vi "Modbus Master Example.vi"() -> ()   [LabVIEW 2016]
doc: "An example of the modbus master functionality."
uses:
  <vilib>/NI/Modbus Library/API/Master/Modbus Master.lvclass
  <vilib>/NI/Modbus Library/API/Wrapper/Create TCP Master.vi
  <vilib>/NI/Modbus Library/API/Wrapper/API Main.lvlib
panel:
  in  "Stop Button":bool
  in  "Port":u16=502
  in  "Set Holding Registers":bool
  in  "Fetch Input Registers":bool
  out "Status":string
  in  "Disconnect":bool
  in  "Connect":bool
  in  "Holding Registers":u16[](array[numeric])=[0, 0, 0, 0, 0, 0, 0, 0]
  out "Input Registers":u16[](array[numeric])
  in  "Slave Address":string="localhost"
  # "Input Registers are the integer inputs of a modbus device. This example allows you to read the first 8 inputs."
  # "Holding Registers are the integer outputs of a modbus device. This example allows you to set the first 8 outputs."
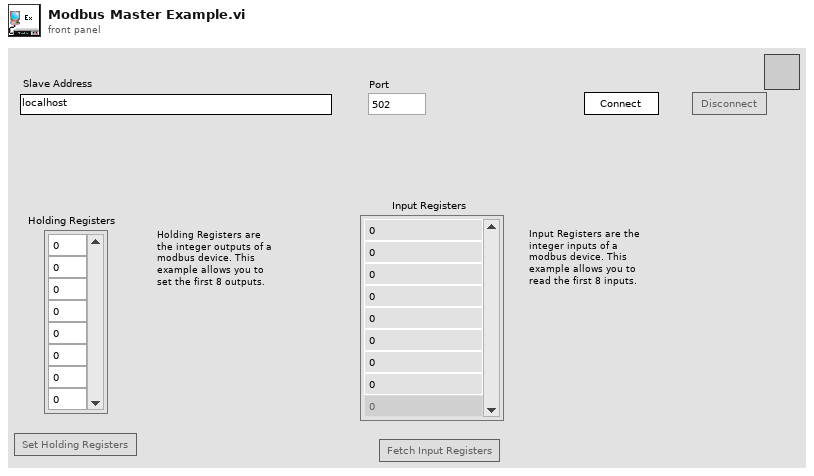
[diagram p1: front panel]
types:
  T1 = enum8{"Enabled", "Disabled", "Disabled and Grayed Out"}
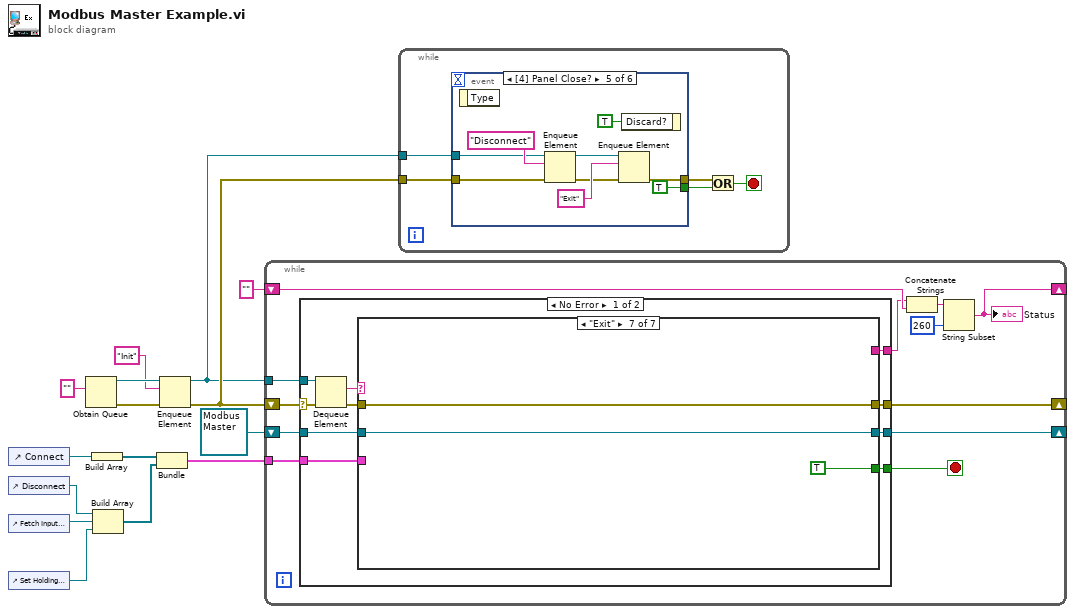
[diagram p0: block diagram]
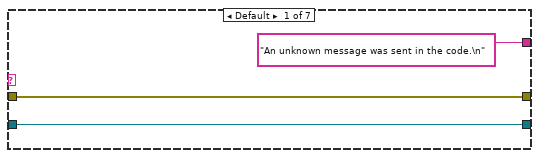
[diagram p2: hidden frame]
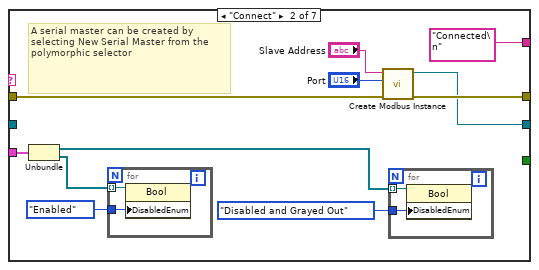
[diagram p3: hidden frame]
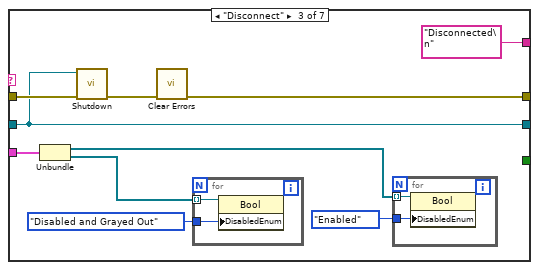
[diagram p4: hidden frame]
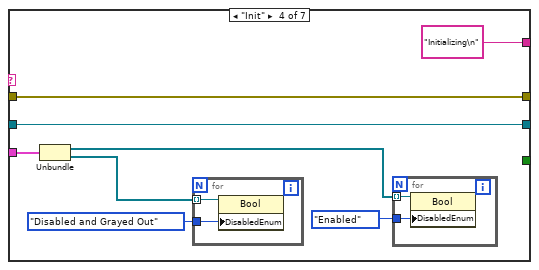
[diagram p5: hidden frame]
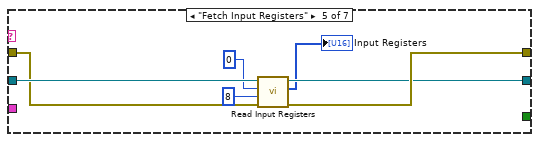
[diagram p6: hidden frame]
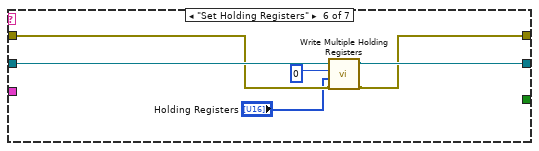
[diagram p7: hidden frame]
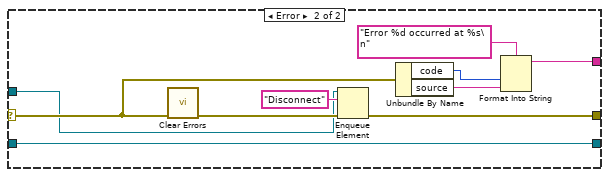
[diagram p8: hidden frame]
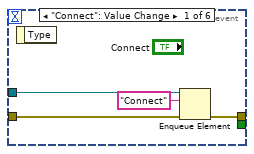
[diagram p9: hidden frame]
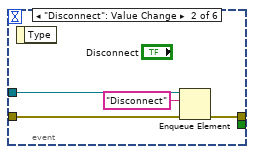
[diagram p10: hidden frame]
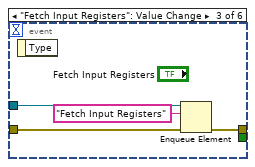
[diagram p11: hidden frame]
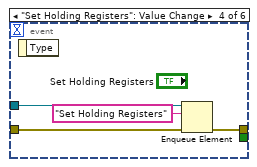
[diagram p12: hidden frame]
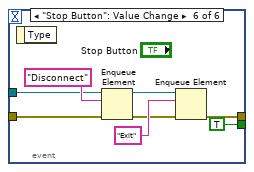
[diagram p13: hidden frame]
diagram:
  n1 = control-ref of="Connect"() -> (w12:refnum<vi>)
  n2 = control-ref of="Disconnect"() -> (w3:refnum<vi>)
  n3 = control-ref of="Fetch Input Registers"() -> (w2:refnum<vi>)
  n4 = control-ref of="Set Holding Registers"() -> (w1:refnum<vi>)
  n5 = Obtain Queue(element data type="") -> (queue out=w7:refnum<queue>, error out=w15:errorcluster)  [unwired: 4 in, 1 out]
  n6 = Build Array(w12) -> (w9:refnum<vi>[])
  n7 = Build Array(w3, w2, w1) -> (w11:refnum<vi>[])
  n8 = Bundle(w9, w11) -> (w10:cluster{refnum<vi>[], refnum<vi>[]})  [unwired: 1 in]
  n9 = Enqueue Element(queue=w7, element="Init", error in (no error)=w15) -> (queue out=w6:refnum<queue>, error out=w8:errorcluster)  [unwired: 1 in, 1 out]
  n10 = while {
    shift-right: [w19] -> _
    shift-left: refnum<class "Modbus Master.lvclass"> refnum ("Modbus Master") -> [w18]
    tunnel: w6 -> [w27]
    shift-right: [w25] -> _
    shift-left: w8 -> [w26]
    shift-right: [w24] -> _
    shift-left: "" ("Status") -> [w21]
    tunnel: w10 -> [w16]
    stop <- w17 stop-if-true
    n11 = case shown="No Error" w26 {
      selector: w26 -> [w36 w105]
      tunnel: w27 -> [w37 w99]
      tunnel: [w33 w106] -> w25
      tunnel: [w30 w102] -> w20
      tunnel: [w32 w98] -> w19
      tunnel: w18 -> [w31 w98]
      tunnel: [w29 _] -> w17
      tunnel: w16 -> [w28 _]
      frame No Error {
        n12 = Dequeue Element(queue=w37, error in (no error)=w36) -> (element=w34:string, error out=w35:errorcluster)  [unwired: 1 in, 2 out]
        n13 = case shown="\"Exit\"" w34 {
          tunnel: w35 -> [w40 w50 w65 w77 w85 w91 w97]
          tunnel: [w40 w49 w61 w77 w88 w92 w97] -> w33
          tunnel: [w39 w48 w63 w76 w87 w93 w96] -> w32
          tunnel: w31 -> [w39 _ w63 w76 w86 w94 w96]
          tunnel: ["An unknown message was sent in the code.\n" "Connected\n" "Disconnected\n" "Initializing\n" _ _ _] -> w30
          tunnel: [_ _ _ _ _ _ TRUE] -> w29
          tunnel: w28 -> [_ w46 w60 w74 _ _ _]
          frame Default {
          }
          frame "Connect" {
            # "A serial master can be created by selecting New Serial Master from the polymorphic selector"
            n14 = Unbundle(w46) -> (w44:refnum<vi>[], w45:refnum<vi>[])
            n15 = for {
              tunnel: w45 -> [w53] mode=indexing
              tunnel: T1."Enabled" ("Disabled") -> [w52]
              n16 = property class="Bool"(reference=w53, "DisabledEnum"=w52) -> ()  [unwired: 1 in, 2 out]
            }
            n17 = call-poly <vilib>:"Create Modbus Instance.vi"("error in"=w50, "port (502)"="Port", "address"="Slave Address") -> ("error out"=w49:errorcluster, "TCP master instance"=w48:refnum<class "Modbus Master.lvclass">)  [unwired: 7 in]
            n18 = for {
              tunnel: w44 -> [w55] mode=indexing
              tunnel: T1."Disabled and Grayed Out" ("Disabled") -> [w54]
              n19 = property class="Bool"(reference=w55, "DisabledEnum"=w54) -> ()  [unwired: 1 in, 2 out]
            }
          }
          frame "Disconnect" {
            n20 = Unbundle(w60) -> (w58:refnum<vi>[], w59:refnum<vi>[])
            n21 = call-dynamic "Shutdown.vi"("error in"=w65, "Modbus master in"=w63) -> ("error out"=w64:errorcluster)  [unwired: 9 in]
            n22 = call <vilib>:"Clear Errors.vi"("error in (no error)"=w64) -> ("error out"=w61:errorcluster)  [unwired: 5 in, 1 out]
            n23 = for {
              tunnel: w59 -> [w69] mode=indexing
              tunnel: T1."Disabled and Grayed Out" ("Disabled") -> [w68]
              n24 = property class="Bool"(reference=w69, "DisabledEnum"=w68) -> ()  [unwired: 1 in, 2 out]
            }
            n25 = for {
              tunnel: w58 -> [w67] mode=indexing
              tunnel: T1."Enabled" ("Disabled") -> [w66]
              n26 = property class="Bool"(reference=w67, "DisabledEnum"=w66) -> ()  [unwired: 1 in, 2 out]
            }
          }
          frame "Init" {
            n27 = Unbundle(w74) -> (w72:refnum<vi>[], w73:refnum<vi>[])
            n28 = for {
              tunnel: w73 -> [w81] mode=indexing
              tunnel: T1."Disabled and Grayed Out" ("Disabled") -> [w80]
              n29 = property class="Bool"(reference=w81, "DisabledEnum"=w80) -> ()  [unwired: 1 in, 2 out]
            }
            n30 = for {
              tunnel: w72 -> [w79] mode=indexing
              tunnel: T1."Enabled" ("Disabled") -> [w78]
              n31 = property class="Bool"(reference=w79, "DisabledEnum"=w78) -> ()  [unwired: 1 in, 2 out]
            }
          }
          frame "Fetch Input Registers" {
            n32 = call-dynamic "Read Input Registers.vi"("error in"=w85, "number of inputs"=u16 8 ("number of registers"), "starting address"=u16 0, "Modbus master in"=w86) -> ("error out"=w88:errorcluster, "register values"=→"Input Registers":u16[], "Modbus master out"=w87:refnum<class "Modbus Master.lvclass">)  [unwired: 5 in]
          }
          frame "Set Holding Registers" {
            n33 = call-dynamic "Write Multiple Holding Registers.vi"("error in"=w91, "registers to write"="Holding Registers", "starting address"=u16 0, "Modbus master in"=w94) -> ("error out"=w92:errorcluster, "Modbus master out"=w93:refnum<class "Modbus Master.lvclass">)  [unwired: 6 in]
          }
          frame "Exit" {
          }
        }
      }
      frame Error {
        n34 = call <vilib>:"Clear Errors.vi"("error in (no error)"=w105) -> ("error out"=w107:errorcluster)  [unwired: 5 in, 1 out]
        n35 = Enqueue Element(queue=w99, element="Disconnect", error in (no error)=w107) -> (error out=w106:errorcluster)  [unwired: 1 in, 2 out]
        n36 = Unbundle By Name(w105) -> ("code"=w104:i32, "source"=w103:string)
        n37 = Format Into String(format string="Error %d occurred at %s\n", w104, w103) -> (resulting string=w102:string)  [unwired: 2 in, 1 out]
      }
    }
    n38 = Concatenate Strings(w20, w21) -> (w22:string)
    n39 = String Subset(string=w22, length (rest)=260 ("length (rest)")) -> (substring=w24:string)  [unwired: 1 in]
    "Status" <- w24
  }
  n40 = while {
    tunnel: w8 -> [w112]
    tunnel: w6 -> [w111]
    stop <- w108 stop-if-true
    n41 = event shown="[4] Panel Close?" {
      selector: _ -> [_ _ _ _ _ _]
      dyn-events: _ -> [_ _ _ _ _ _]
      timeout: _ -> [_ _ _ _ _ _]
      tunnel: w112 -> [w116 w120 w124 w128 w134 w143]
      tunnel: [w115 w119 w123 w127 w129 w138] -> w110
      tunnel: w111 -> [w114 w118 w122 w126 w131 w140]
      tunnel: [_ _ _ _ TRUE ("Discard?") TRUE ("Discard?")] -> w109
      event "Connect": Value Change {
        n42 = event-data() -> ()  [unwired: 1 in, 1 out]
        n43 = Enqueue Element(queue=w114, element="Connect", error in (no error)=w116) -> (error out=w115:errorcluster)  [unwired: 1 in, 2 out]
      }
      event "Disconnect": Value Change {
        n44 = event-data() -> ()  [unwired: 1 in, 1 out]
        n45 = Enqueue Element(queue=w118, element="Disconnect", error in (no error)=w120) -> (error out=w119:errorcluster)  [unwired: 1 in, 2 out]
      }
      event "Fetch Input Registers": Value Change {
        n46 = event-data() -> ()  [unwired: 1 in, 1 out]
        n47 = Enqueue Element(queue=w122, element="Fetch Input Registers", error in (no error)=w124) -> (error out=w123:errorcluster)  [unwired: 1 in, 2 out]
      }
      event "Set Holding Registers": Value Change {
        n48 = event-data() -> ()  [unwired: 1 in, 1 out]
        n49 = Enqueue Element(queue=w126, element="Set Holding Registers", error in (no error)=w128) -> (error out=w127:errorcluster)  [unwired: 1 in, 2 out]
      }
      event Panel Close? {
        n50 = event-data() -> ()  [unwired: 1 in, 1 out]
        n51 = Enqueue Element(queue=w131, element="Disconnect", error in (no error)=w134) -> (queue out=w132:refnum<queue>, error out=w130:errorcluster)  [unwired: 1 in, 1 out]
        n52 = Enqueue Element(queue=w132, element="Exit", error in (no error)=w130) -> (error out=w129:errorcluster)  [unwired: 1 in, 2 out]
        n53 = event-data("Discard?"=TRUE) -> ()  [unwired: 1 in, 1 out]
      }
      event "Stop Button": Value Change {
        n54 = event-data() -> ()  [unwired: 1 in, 1 out]
        n55 = Enqueue Element(queue=w140, element="Disconnect", error in (no error)=w143) -> (queue out=w141:refnum<queue>, error out=w139:errorcluster)  [unwired: 1 in, 1 out]
        n56 = Enqueue Element(queue=w141, element="Exit", error in (no error)=w139) -> (error out=w138:errorcluster)  [unwired: 1 in, 2 out]
      }
    }
    n57 = Or(x=w110, y=w109) -> (x .or. y?=w108:bool)
  }
